vi "generate table.vi"(0 "TEC in":refnum<class "TEC configuration.lvclass">, 1 "from TEC":refnum<vi>, 2 "to TEC":refnum<vi>, 3 "avail tags":refnum<vi>, 5 "Pair in":refnum<class "TEC configuration.lvclass">, 7 "engine configuration in":refnum<class "engine configuration.lvclass">, 9 "paired engine in":refnum<class "engine configuration.lvclass">, 11 "error in":errorcluster) -> (4 "TEC out":refnum<class "TEC configuration.lvclass">, 6 "pair out":refnum<class "TEC configuration.lvclass">, 8 "engine configuration out":refnum<class "engine configuration.lvclass">, 10 "paired engine out":refnum<class "engine configuration.lvclass">, 15 "error out":errorcluster)   [LabVIEW 2013, in "TEC editor node.lvclass"]
uses:
  TEC editor node.lvclass
  configuration/TEC configuration.lvclass
  <vilib>/NI/Module Execution Interface/Engine Configuration/engine configuration.lvclass
  <vilib>/NI/Tag Bus Module Framework/channel/channel classification.ctl
  <vilib>/NI/Tag Bus/tag/tag descriptor.lvclass/tag descriptor.ctl
  <vilib>/NI/Configuration Framework/serializable configuration/NISE_CEF_serializable configuration.lvclass/NISE_CEF_serializable configuration.ctl
  <vilib>/NI/Configuration Framework/serializable configuration/NISE_CEF_serializable configuration.lvclass
  <vilib>/NI/Module Execution Interface/Engine Configuration/engine configuration.lvclass/engine configuration.ctl
  <vilib>/NI/Tag Bus/tag/tag descriptor.lvclass
  <vilib>/NI/Tag Bus Module Framework/channel/TBM channel.lvclass
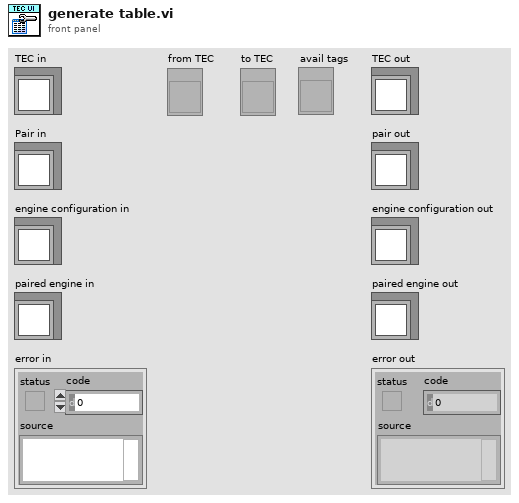
[diagram p1: front panel]
types:
  T1 = typedef "TBM channel.lvclass/channel classification.ctl" = enum16{"input data", "output data", "processing parameter", "processing result"}
  T2 = typedef "tag bus.lvlib/tag descriptor.lvclass/Data Type.ctl" = enum16{"Double", "Single", "I64", "I32", "I16", "I8", "U64", "U32", "U16", "U8", "Boolean", "String", "Array of Double", "Array of Single", "Array of I64", "Array of I32", "Array of I16", "Array of I8", "Array of U64", "Array of U32", "Array of U16", "Array of U8", "Array of Boolean", "Array of String"}
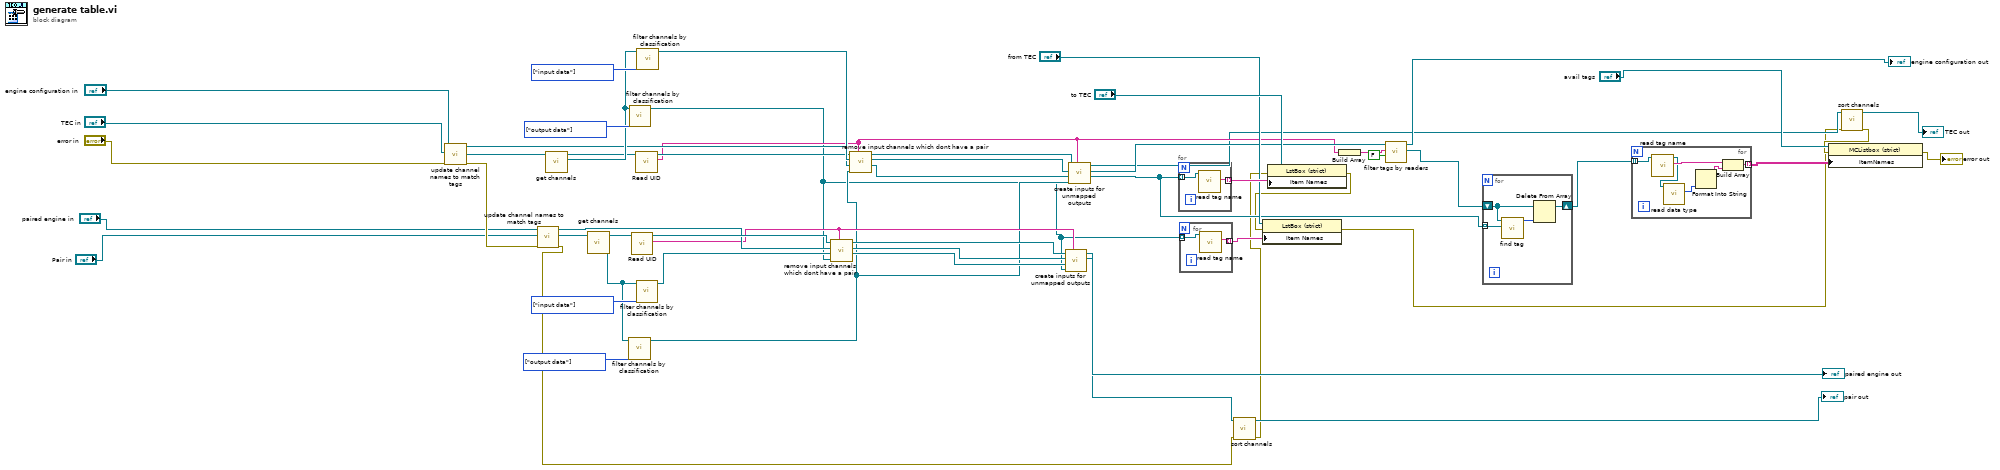
[diagram p0: block diagram]
diagram:
  w45 = T1[] [enum."output data"] items=["input data", "output data", "processing parameter", "processing result"] ("allowed classifications")
  w44 = T1[] [enum."input data"] items=["input data", "output data", "processing parameter", "processing result"] ("allowed classifications")
  w47 = T1[] [enum."output data"] items=["input data", "output data", "processing parameter", "processing result"] ("allowed classifications")
  w48 = T1[] [enum."input data"] items=["input data", "output data", "processing parameter", "processing result"] ("allowed classifications")
  n1 = call "update channel names to match tags.vi"("error in"="error in", "TEC in"="TEC in", "engine configuration in"="engine configuration in") -> ("error out"=w53:errorcluster, "TEC out"=w50:refnum<class "TEC configuration.lvclass">, "engine configuration out"=w42:refnum<class "engine configuration.lvclass">)  [unwired: 6 in]
  n2 = call "update channel names to match tags.vi"("error in"=w53, "TEC in"="Pair in", "engine configuration in"="paired engine in") -> ("error out"=w5:errorcluster, "TEC out"=w49:refnum<class "TEC configuration.lvclass">, "engine configuration out"=w35:refnum<class "engine configuration.lvclass">)  [unwired: 6 in]
  n3 = call-dynamic "get channels.vi"("TEC configuration in"=w50) -> ("channels"=w43:refnum<class "TBM channel.lvclass">[], "TEC configuration out"=w40:refnum<class "TEC configuration.lvclass">)  [unwired: 9 in]
  n4 = call-dynamic "get channels.vi"("TEC configuration in"=w49) -> ("channels"=w46:refnum<class "TBM channel.lvclass">[], "TEC configuration out"=w38:refnum<class "TEC configuration.lvclass">)  [unwired: 9 in]
  n5 = call <vilib>:"filter channels by classification.vi"("allowed classifications"=w47, "channels in"=w46) -> ("channels out"=w15:refnum<class "TBM channel.lvclass">[])  [unwired: 9 in]
  n6 = call <vilib>:"filter channels by classification.vi"("allowed classifications"=w45, "channels in"=w43) -> ("channels out"=w14:refnum<class "TBM channel.lvclass">[])  [unwired: 9 in]
  n7 = call <vilib>:"Read UID.vi"("configuration in"=w38) -> ("instance id"=w16:string, "configuration out"=w36:refnum<class "TEC configuration.lvclass">)  [unwired: 8 in, 1 out]
  n8 = call <vilib>:"Read UID.vi"("configuration in"=w40) -> ("instance id"=w17:string, "configuration out"=w39:refnum<class "TEC configuration.lvclass">)  [unwired: 8 in, 1 out]
  n9 = call <vilib>:"filter channels by classification.vi"("allowed classifications"=w48, "channels in"=w46) -> ("channels out"=w37:refnum<class "TBM channel.lvclass">[])  [unwired: 9 in]
  n10 = call <vilib>:"filter channels by classification.vi"("allowed classifications"=w44, "channels in"=w43) -> ("channels out"=w41:refnum<class "TBM channel.lvclass">[])  [unwired: 9 in]
  n11 = call "remove input channels which dont have a pair.vi"("instance id"=w16, "output channels"=w14, "input channels"=w37, "engine configuration in"=w35, "TEC configuration in"=w36) -> ("input channels out"=w29:refnum<class "TBM channel.lvclass">[], "engine configuration out"=w30:refnum<class "engine configuration.lvclass">, "TEC configuration out"=w31:refnum<class "TEC configuration.lvclass">)  [unwired: 4 in]
  n12 = call "remove input channels which dont have a pair.vi"("instance id"=w17, "output channels"=w15, "input channels"=w41, "engine configuration in"=w42, "TEC configuration in"=w39) -> ("input channels out"=w32:refnum<class "TBM channel.lvclass">[], "engine configuration out"=w33:refnum<class "engine configuration.lvclass">, "TEC configuration out"=w34:refnum<class "TEC configuration.lvclass">)  [unwired: 4 in]
  n13 = call "create inputs for unmapped outputs.vi"("module instance"=w16, "outputs"=w14, "input channels in"=w29, "engine configuration in"=w30, "TEC configuration in"=w31) -> ("engine configuration out"=→"paired engine out":refnum<class "engine configuration.lvclass">, "TEC configuration out"=w8:refnum<class "TEC configuration.lvclass">)  [unwired: 4 in, 1 out]
  n14 = call "create inputs for unmapped outputs.vi"("module instance"=w17, "outputs"=w15, "input channels in"=w32, "engine configuration in"=w33, "TEC configuration in"=w34) -> ("input channels out"=w11:refnum<class "TBM channel.lvclass">[], "engine configuration out"=w24:refnum<class "engine configuration.lvclass">, "TEC configuration out"=w10:refnum<class "TEC configuration.lvclass">)  [unwired: 4 in]
  n15 = for {
    tunnel: w11 -> [w58] mode=indexing
    tunnel: [w57] -> w27 mode=indexing
    n16 = call <vilib>:"read tag name.vi"("system tag in"=w58) -> ("name"=w57:string)  [unwired: 8 in, 2 out]
  }
  n17 = for {
    tunnel: w14 -> [w60] mode=indexing
    tunnel: [w59] -> w26 mode=indexing
    n18 = call <vilib>:"read tag name.vi"("system tag in"=w60) -> ("name"=w59:string)  [unwired: 8 in, 2 out]
  }
  n19 = call "sort channels.vi"("error in"=w5, "UDP Broadcaster Configuration in"=w8) -> ("error out"=w3:errorcluster, "UDP Broadcaster Configuration out"=→"pair out":refnum<class "TEC configuration.lvclass">)  [unwired: 8 in]
  n20 = property class="LstBox (strict)"(reference="to TEC", error in=w3, "Item Names"=w27) -> (error out=w2:errorcluster)  [unwired: 1 out]
  n21 = property class="LstBox (strict)"(reference="from TEC", error in=w2, "Item Names"=w26) -> (error out=w1:errorcluster)  [unwired: 1 out]
  n22 = Build Array(w17) -> (w23:string[])
  n23 = call <vilib>:"filter tags by readers.vi"("include? (default: exclude)"=FALSE, "reader modules"=w23, "engine configuration in"=w24) -> ("tag list"=w13:refnum<class "tag descriptor.lvclass">[], "engine configuration out"=→"engine configuration out":refnum<class "engine configuration.lvclass">)  [unwired: 7 in]
  n24 = for {
    shift-right: [w63] -> w12
    shift-left: w13 -> [w64]
    tunnel: w11 -> [w61] mode=indexing
    n25 = call <vilib>:"find tag.vi"("tag"=w61, "tags in"=w64) -> ("index"=w62:i32)  [unwired: 9 in]
    n26 = Delete From Array(array=w64, index=w62) -> (array with subset deleted=w63:refnum<class "tag descriptor.lvclass">[])  [unwired: 1 in, 1 out]
  }
  n27 = for {
    tunnel: w12 -> [w70] mode=indexing
    tunnel: [w66] -> w21 mode=indexing
    n28 = call <vilib>:"read tag name.vi"("system tag in"=w70) -> ("name"=w69:string, "system tag out"=w68:refnum<class "tag descriptor.lvclass">)  [unwired: 8 in, 1 out]
    n29 = call <vilib>:"read data type.vi"("system tag in"=w68) -> ("data type"=w67:T2)  [unwired: 8 in, 2 out]
    n30 = Format Into String(w67) -> (resulting string=w65:string)  [unwired: 3 in, 1 out]
    n31 = Build Array(w69, w65) -> (w66:string[])
  }
  n32 = call "sort channels.vi"("error in"=w1, "UDP Broadcaster Configuration in"=w10) -> ("error out"=w6:errorcluster, "UDP Broadcaster Configuration out"=→"TEC out":refnum<class "TEC configuration.lvclass">)  [unwired: 8 in]
  n33 = property class="MCListbox (strict)"(reference="avail tags", error in=w6, "ItemNames"=w21) -> (error out=→"error out":errorcluster)  [unwired: 1 out]
